vi "Write channel type.vi"(8 "error in (no error)":errorcluster, 10 "channel type":string, 11 "Channel group in":refnum<class "Channel group.lvclass">) -> (0 "error out":errorcluster, 3 "Channel group out":refnum<class "Channel group.lvclass">)   [LabVIEW 2016, in "FPGA RM Shared API.lvlib" / "Channel group.lvclass"]
uses:
  Channel group.lvclass
  Channel group.lvclass/Channel group.ctl
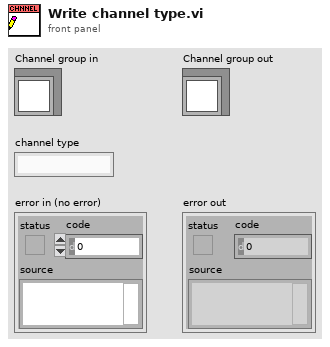
[diagram p1: front panel]
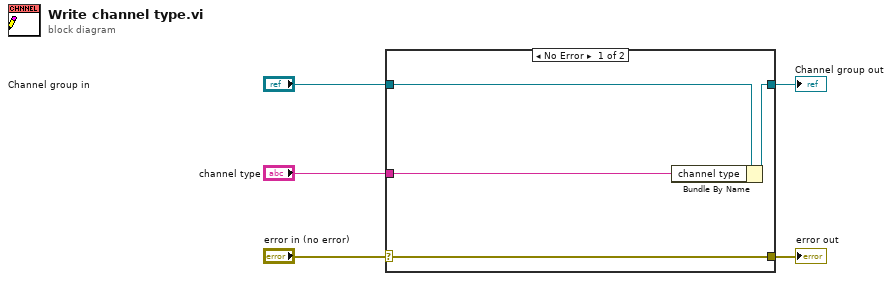
[diagram p0: block diagram]
diagram:
  n1 = case shown="No Error" "error in (no error)" {
    selector: "error in (no error)" -> [w9 w10]
    tunnel: [w9 w10] -> w4
    tunnel: [w7 w11] -> w2
    tunnel: "Channel group in" -> [w8 w11]
    tunnel: "channel type" -> [w6 _]
    frame No Error {
      n2 = Bundle By Name(cluster=w8, "channel type"=w6) -> (w7:refnum<class "Channel group.lvclass">)
    }
    frame Error {
    }
  }
  "error out" <- w4
  "Channel group out" <- w2
